vi "CarregarConfig.vi"(0 "caminho in":path, 5 "error in (no error)":errorcluster) -> (14 "caminho out":path, 15 "DadosCanais":T2[](array[typedef]), 16 "Estaticos":string[][](array[string]), 17 "ConfigSistema":T1, 19 "error out":errorcluster)   [LabVIEW 2017]
uses:
  Typedefs/Tipo_DadosCanal.ctl
  Typedefs/Tipo_TipoSinalSimulado.ctl
  Typedefs/Tipo_ConfigSistema.ctl
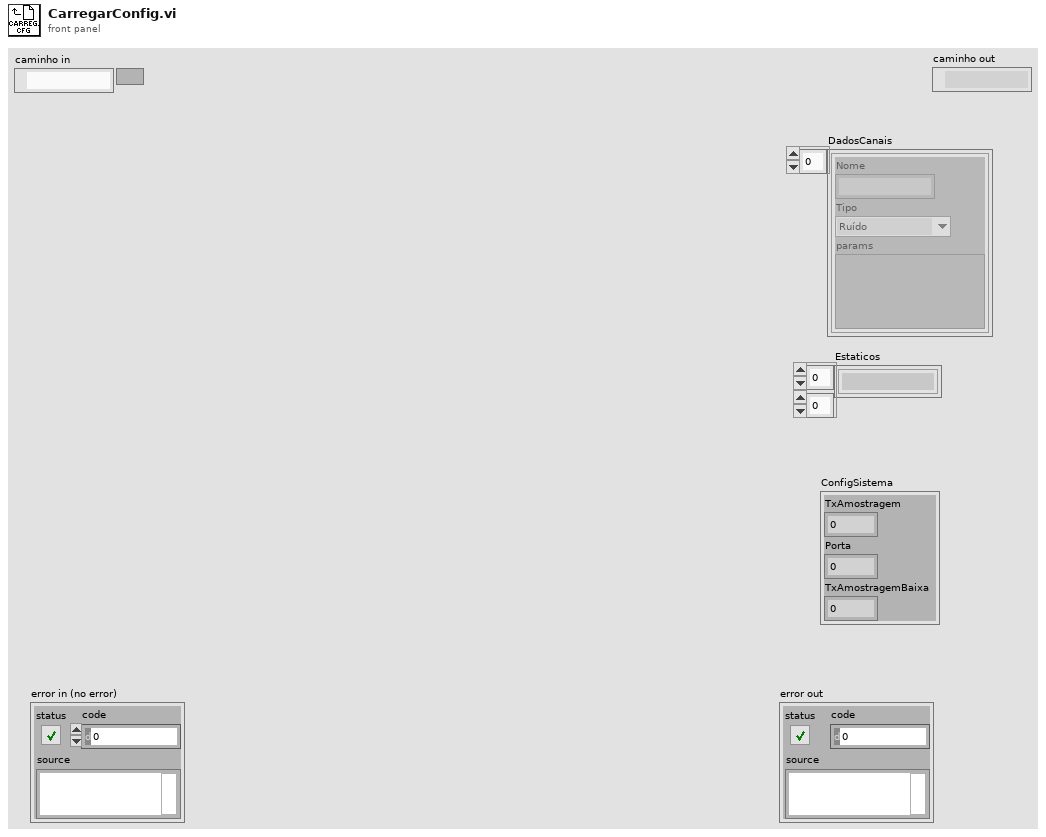
[diagram p1: front panel]
types:
  T1 = typedef "Tipo_ConfigSistema.ctl" = cluster{"TxAmostragem":dbl, "Porta":u16, "TxAmostragemBaixa":dbl}
  T2 = typedef "Tipo_DadosCanal.ctl" = cluster{"Nome":string, "Tipo":T3, "params":variant}
  T3 = typedef "Tipo_TipoSinalSimulado.ctl" = enum16{"Ruído", "Fasor", "Senóide", "Composto", "AM", "Proximidade", "Entreferro"}
  T4 = enum16{"open", "replace", "create", "open or create", "replace or create", "replace or create with confirmation"}
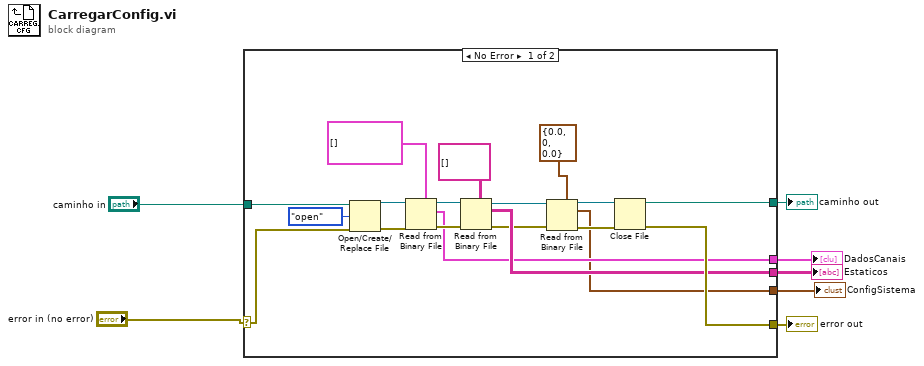
[diagram p0: block diagram]
diagram:
  n1 = case shown="No Error" "error in (no error)" {
    selector: "error in (no error)" -> [w15 w27]
    tunnel: [w26 w27] -> w7
    tunnel: "caminho in" -> [w24 w28]
    tunnel: [w22 _] -> w5
    tunnel: [w19 _] -> w4
    tunnel: [w14 w28] -> w2
    tunnel: [w8 _] -> w1
    frame No Error {
      n2 = Open/Create/Replace File(file path (use dialog)=w24, error in=w15, operation (0:open)=T4."open") -> (refnum out=w18:refnum<file>, error out=w17:errorcluster)  [unwired: 3 in, 1 out]
      n3 = Read from Binary File(5:T2[] [] ("DadosCanais"), 8:w17, 11:w18) -> (0:w23:errorcluster, 2:w19:T2[], 3:w20:refnum<file>)  [unwired: 3 in, 1 out]
      n4 = Read from Binary File(5:string[][] [] ("Item Names"), 8:w23, 11:w20) -> (0:w12:errorcluster, 2:w22:string[][], 3:w13:refnum<file>)  [unwired: 3 in, 1 out]
      n5 = Read from Binary File(5:T1 {"TxAmostragem"=0.0, "Porta"=0, "TxAmostragemBaixa"=0.0} ("output cluster"), 8:w12, 11:w13) -> (0:w11:errorcluster, 2:w8:T1, 3:w10:refnum<file>)  [unwired: 3 in, 1 out]
      n6 = Close File(refnum=w10, error in=w11) -> (path=w14:path, error out=w26:errorcluster)
    }
    frame Error {
    }
  }
  "error out" <- w7
  "Estaticos" <- w5
  "DadosCanais" <- w4
  "caminho out" <- w2
  "ConfigSistema" <- w1
